vi "纳清DO_所有参数读取.vi"(7 "盐度补偿":dbl, 8 "error in (no error)":errorcluster caption="错误输入（无错误）", 11 "MB session in":refnum<class "MB_Master.lvclass">) -> (0 "error out":errorcluster caption="错误输出", 2 "输出值":T1 {"波特率" items=["4800", "9600", "19200", "38400", "57600", "115200"]}, 3 "MB session out":refnum<class "MB_Master.lvclass">)   [LabVIEW 2016, in "斯坦道多参数.lvlib"]
uses:
  <vilib>/Plasmionique/MB Master/MB_Master/MB_Master.lvclass
  <vilib>/Plasmionique/MB Master/MB Master.lvlib
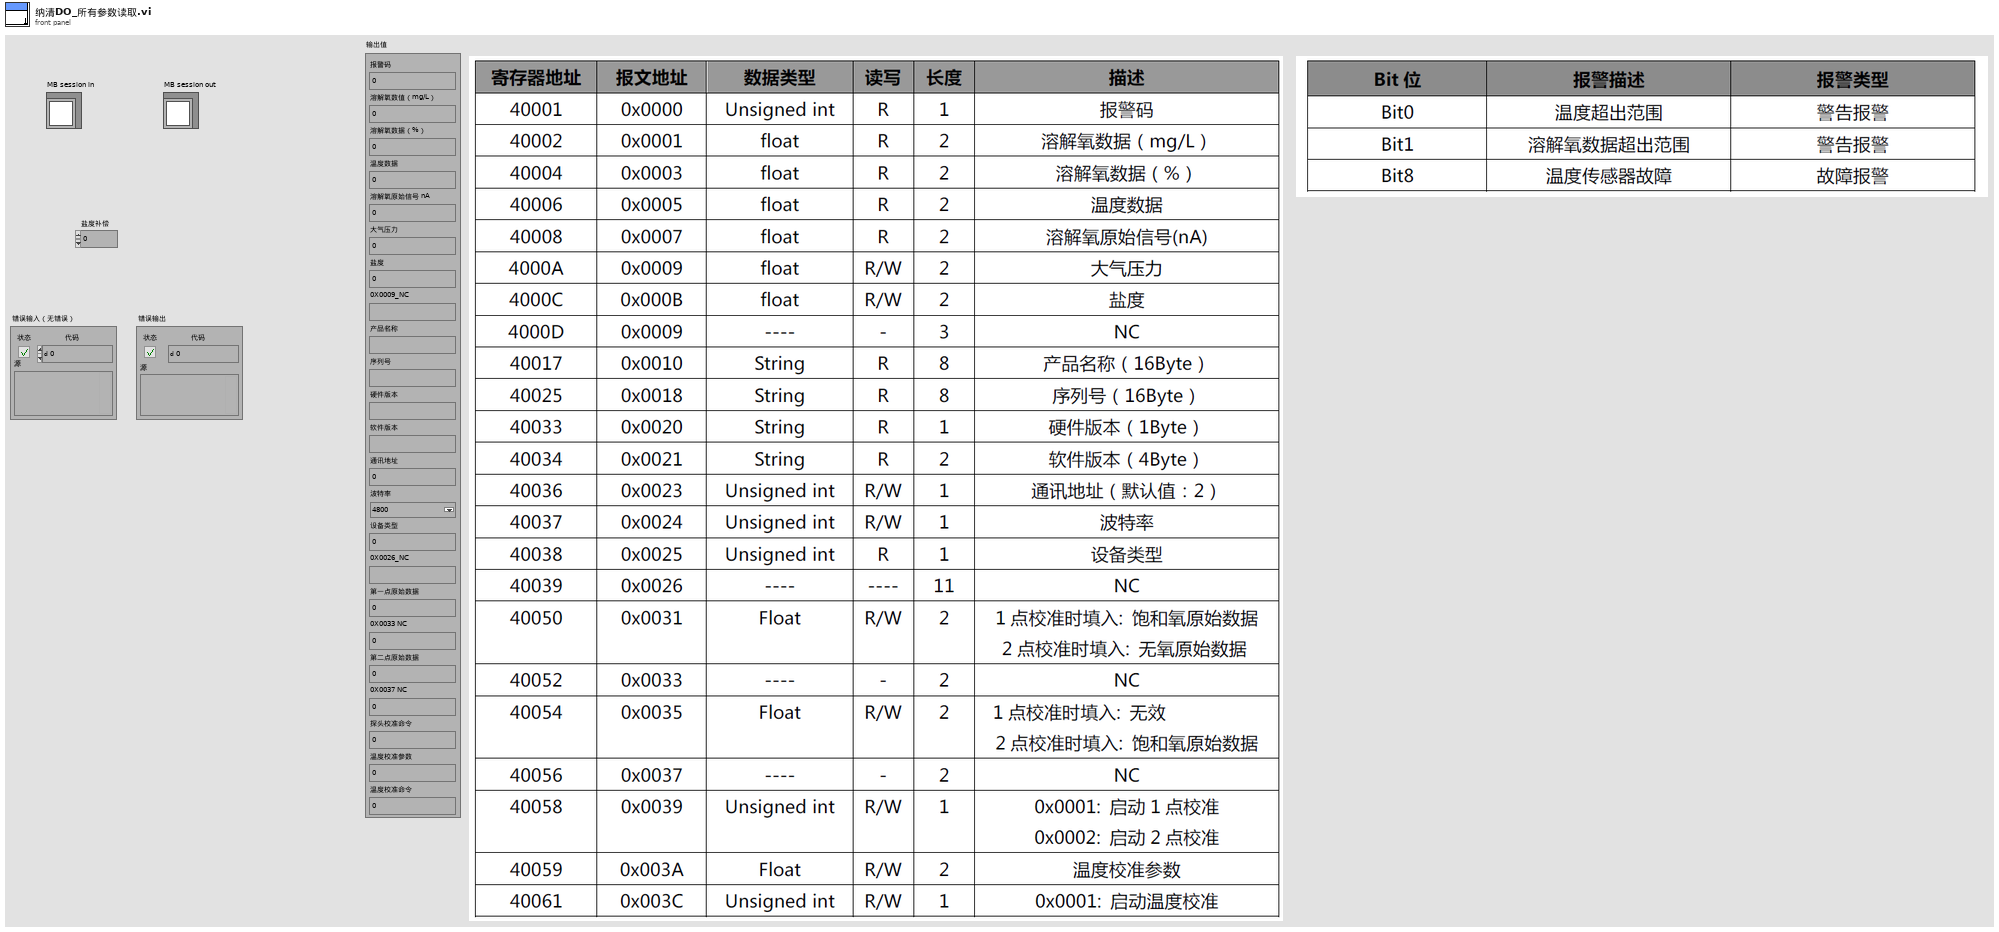
[diagram p1: front panel]
types:
  T1 = cluster{"报警码":u16, "溶解氧数值（mg/L）":sgl, "溶解氧数据（%）":sgl, "温度数据":sgl, "溶解氧原始信号 nA":sgl, "大气压力":sgl, "盐度":sgl, "0X0009_NC":string, "产品名称":string, "序列号":string, "硬件版本":string, "软件版本":string, "通讯地址":u16, "波特率":u16, "设备类型":u16, "0X0026_NC":string, "第一点原始数据":sgl, "0X0033 NC":sgl, "第二点原始数据":sgl, "0X0037 NC":sgl, "探头校准命令":u16, "温度校准参数":sgl, "温度校准命令":u16}
  T2 = cluster{"pH":u32, "DO":u32, "Cond":u32, "Turb":u32, "叶绿素a":u32, "藻密度":u32, "ORP":u32}
  T3 = cluster{u16, "mode":dbl, "数值":sgl, "数值":sgl, "数值":sgl, "数值":sgl, "盐度补偿":dbl, "类型":string, "类型":string, "类型":string, "类型":string, "类型":string, u16, u16, u16, "类型":string, "数值":sgl, "数值":sgl, "数值":sgl, "数值":sgl, u16, "数值":sgl, u16}
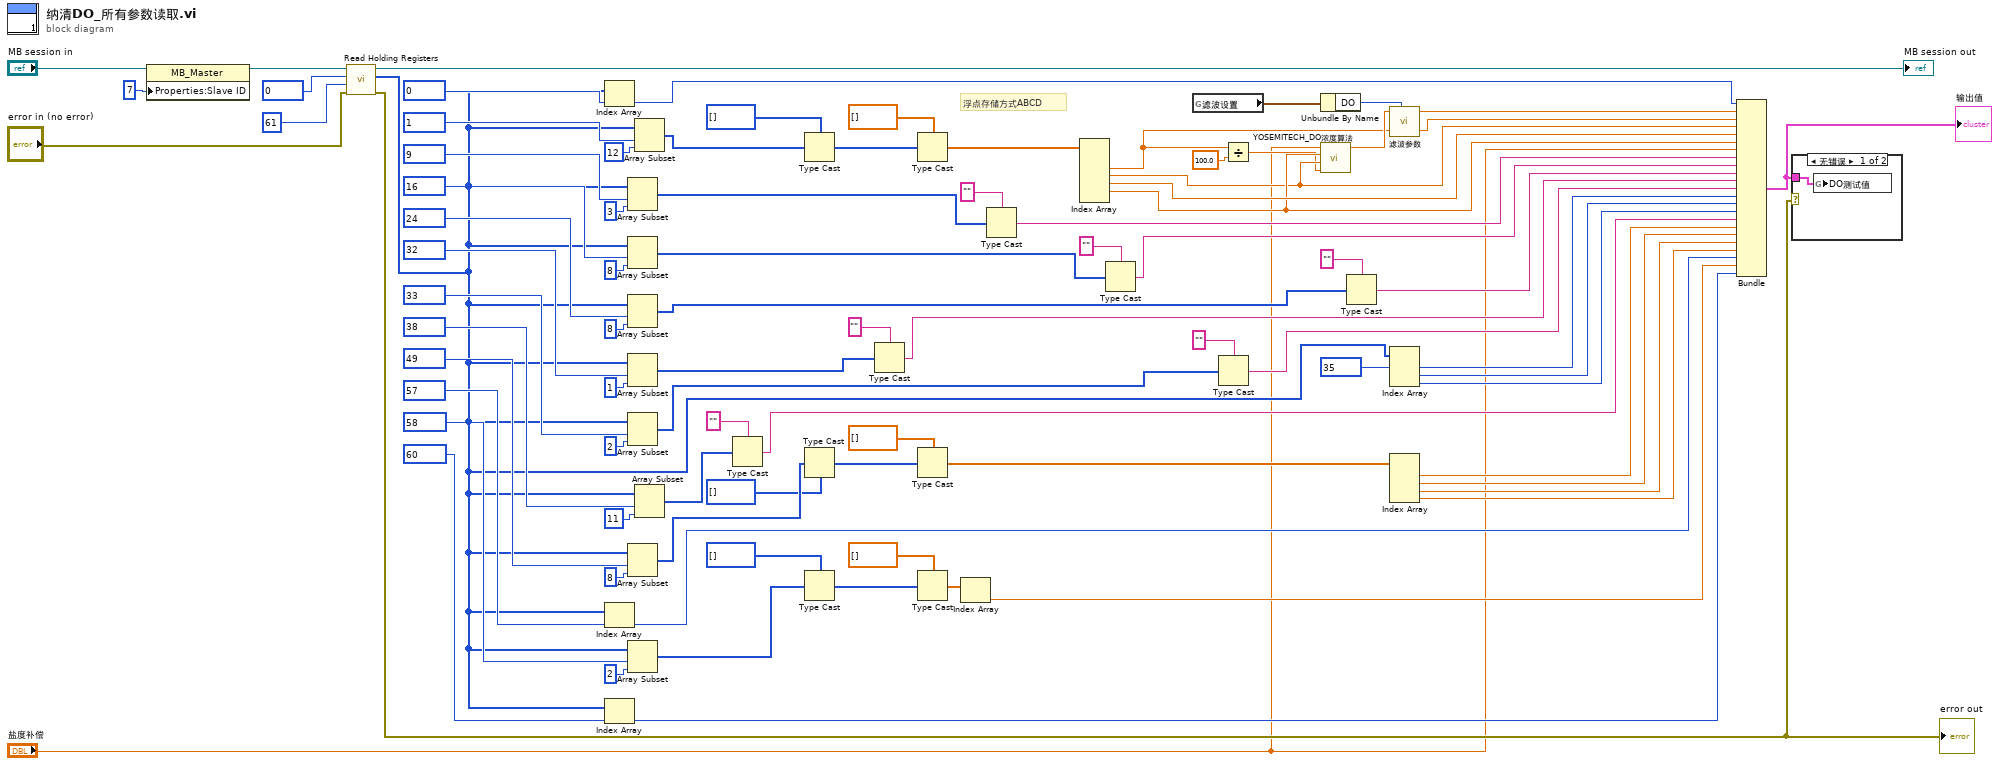
[diagram p0: block diagram]
diagram:
  # "浮点存储方式ABCD"
  n1 = property class="MB_Master"(reference="MB session in", "Properties:Slave ID"=u8 7 ("Slave ID")) -> (reference out=w77:refnum<class "MB_Master.lvclass">)  [unwired: 1 in, 1 out]
  n2 = call <vilib>:"Read Holding Registers.vi"("error in (no error)"="error in (no error)", "quantity"=u16 61, "starting address"=u16 0, "MB session in"=w77) -> ("error out"=w19:errorcluster, "Registers"=w21:u16[], "MB session out"=→"MB session out":refnum<class "MB_Master.lvclass">)  [unwired: 5 in]
  "error out" <- w19
  n3 = Index Array(array=w21, index=u16 0 ("starting address")) -> (element=w85:u16)
  n4 = Index Array(array=w21, index=u16 57 ("starting address")) -> (element=w24:u16)
  n5 = Index Array(array=w21, index=u16 60 ("starting address")) -> (element=w20:u16)
  n6 = Array Subset(array=w21, index=u16 9 ("starting address"), length=3 ("长度")) -> (w72:u16[])
  n7 = Array Subset(array=w21, index=u16 16 ("starting address"), length=8 ("长度")) -> (w68:u16[])
  n8 = Array Subset(array=w21, index=u16 24 ("starting address"), length=8 ("长度")) -> (w62:u16[])
  n9 = Array Subset(array=w21, index=u16 32 ("starting address"), length=1 ("长度")) -> (w58:u16[])
  n10 = Array Subset(array=w21, index=u16 33 ("starting address"), length=2 ("长度")) -> (w52:u16[])
  n11 = Array Subset(array=w21, index=u16 49 ("starting address"), length=8 ("长度")) -> (w39:u16[])
  n12 = Array Subset(array=w21, index=u16 58 ("starting address"), length=2 ("长度")) -> (w27:u16[])
  n13 = Array Subset(array=w21, index=u16 1 ("starting address"), length=12 ("长度")) -> (w81:u16[])
  n14 = Array Subset(array=w21, index=u16 38 ("starting address"), length=11 ("长度")) -> (w42:u16[])
  n15 = Type Cast(type="" ("类型"), x=w42) -> (*(type *) &x=w41:string)
  n16 = Type Cast(type=u32[] [] ("数组 2"), x=w81) -> (*(type *) &x=w18:u32[])
  n17 = Type Cast(type=u32[] [] ("数组 2"), x=w39) -> (*(type *) &x=w37:u32[])
  n18 = Type Cast(type=u32[] [] ("数组 2"), x=w27) -> (*(type *) &x=w29:u32[])
  n19 = Type Cast(type="" ("类型"), x=w58) -> (*(type *) &x=w55:string)
  n20 = Type Cast(type=sgl[] [] ("数组 2"), x=w18) -> (*(type *) &x=w80:sgl[])
  n21 = Type Cast(type=sgl[] [] ("数组 2"), x=w37) -> (*(type *) &x=w34:sgl[])
  n22 = Type Cast(type=sgl[] [] ("数组 2"), x=w29) -> (*(type *) &x=w32:sgl[])
  n23 = Index Array(array=w32) -> (element=w23:sgl)  [unwired: 1 in]
  n24 = Type Cast(type="" ("类型"), x=w72) -> (*(type *) &x=w70:string)
  n25 = Index Array(array=w80) -> (element #2=w4:sgl, element #3=w6:sgl, element #4=w15:sgl, element #5=w7:sgl)  [unwired: 6 in, 2 out]
  n26 = Type Cast(type="" ("类型"), x=w68) -> (*(type *) &x=w65:string)
  n27 = global read "断电保存变量.vi" "滤波设置"() -> (w9:T2)
  n28 = Type Cast(type="" ("类型"), x=w52) -> (*(type *) &x=w50:string)
  n29 = Divide(x=w4, y=sgl 100.0) -> (x/y=w2:sgl)
  n30 = Unbundle By Name(w9) -> ("DO"=w8:u32)
  n31 = call "YOSEMITECH_DO浓度算法.vi"("溶解氧饱和度值"=w2, "水温"=w6, "大气压补偿"=w7, "盐度补偿"="盐度补偿") -> ("DataDo_mgL"=w5:dbl)  [unwired: 7 in]
  n32 = Type Cast(type="" ("类型"), x=w62) -> (*(type *) &x=w60:string)
  n33 = call "滤波参数.vi"("滤波次数"=w8, "x"=w5) -> ("mode"=w10:dbl)  [unwired: 9 in]
  n34 = Index Array(array=w21, index #1=u16 35 ("starting address")) -> (element #1=w48:u16, element #2=w47:u16, element #3=w46:u16)  [unwired: 2 in]
  n35 = Index Array(array=w34) -> (element #1=w33:sgl, element #2=w14:sgl, element #3=w13:sgl, element #4=w12:sgl)  [unwired: 4 in]
  n36 = Bundle(w85, "mode"=w10, "数值"=w4, "数值"=w6, "数值"=w15, "数值"=w7, "盐度补偿"="盐度补偿", "类型"=w70, "类型"=w65, "类型"=w60, "类型"=w55, "类型"=w50, w48, w47, w46, "类型"=w41, "数值"=w33, "数值"=w14, "数值"=w13, "数值"=w12, w24, "数值"=w23, w20) -> (w11:T3)  [unwired: 1 in]
  "输出值" <- w11
  n37 = case shown="无错误" w19 {
    tunnel: w11 -> [w88 _]
    frame No Error {
      n38 = global write "纳清过程全局变量.vi" "DO测试值"(w88) -> ()
    }
    frame Error {
    }
  }
